vi "Insert in Cache (element).vi"(9 "element":string, 10 "key":string, 11 "xml cache in":T1) -> (2 "element not found?":bool, 3 "xml cache out":T1)   [LabVIEW 2020, in "Configuration_Helper.lvlib"]
uses:
  Configuration_Helper.lvlib
  <vilib>/Utility/miscctls.llb/LVMapReplaceAction.ctl
  _typedefs/xml_1553_cache_type.ctl
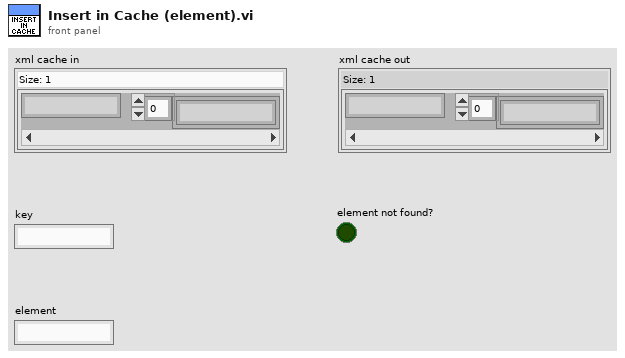
[diagram p1: front panel]
types:
  T1 = typedef "Configuration_Helper.lvlib/xml_1553_cache_type.ctl" = map{string, string[]}
  T2 = typedef "LVMapReplaceAction.ctl" = enum32{"Modify Entry only if found", "Add or Modify Entry", "Delete Entry"}
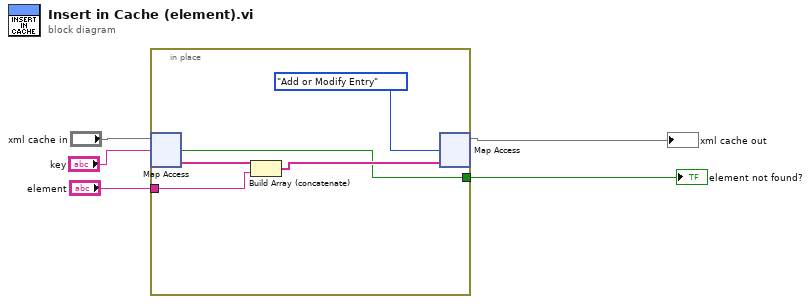
[diagram p0: block diagram]
diagram:
  n1 = in-place {
    in-place-border: "element" -> [w7]
    in-place-border: [w6] -> w1
    n2 = in-place-map #1("xml cache in", "key") -> (w10:string[], w6:bool)  [unwired: 1 in]
    n3 = Build Array (concatenate)(w10, w7) -> (w9:string[])
    n4 = in-place-map #1(w9, LVMapReplaceAction."Add or Modify Entry" ("action")) -> (→"xml cache out":T1)  [unwired: 2 out]
  }
  "element not found?" <- w1
